vi "YokoGS200 Set Levelold.vi"(8 "error in (no error)":errorcluster, 9 "Auto Range":bool, 10 "Output Level":dbl min=-30.0 max=30.0 step=1e-08, 11 "VISA Rsrc":refnum<visa-resource-name>="SR530") -> (0 "error out":errorcluster, 3 "VISA Rsrc Out":refnum<visa-resource-name>="GPIB0::12::INSTR")   [LabVIEW 2012]
uses:
  <userlib>/Yoko GS200/YokoGS200 lvl_states ctl.ctl
panel:
  out "Octet d'état":bool[](array[boolean])
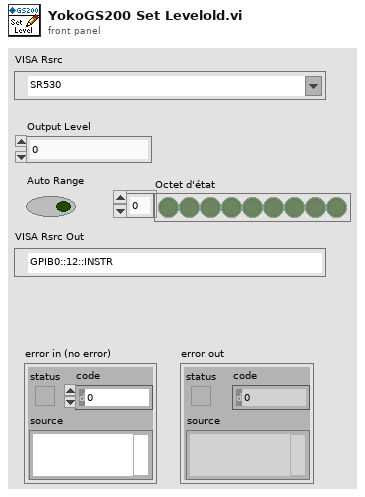
[diagram p1: front panel]
types:
  T1 = typedef "YokoGS200 lvl_states ctl.ctl" = enum16{"Send Command", "Check Errors", "End"}
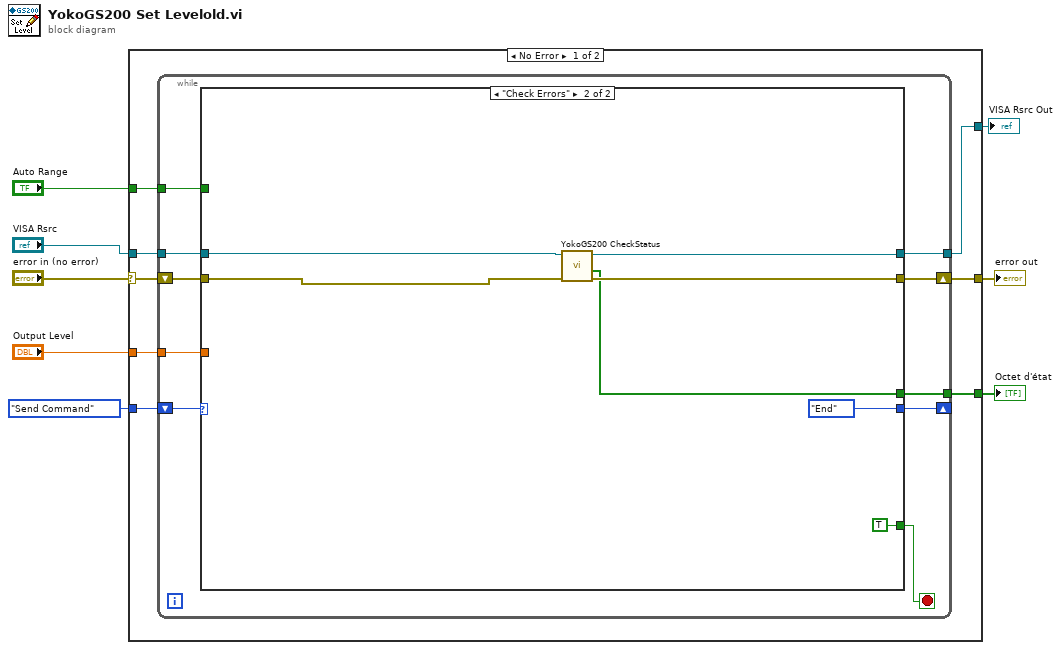
[diagram p0: block diagram]
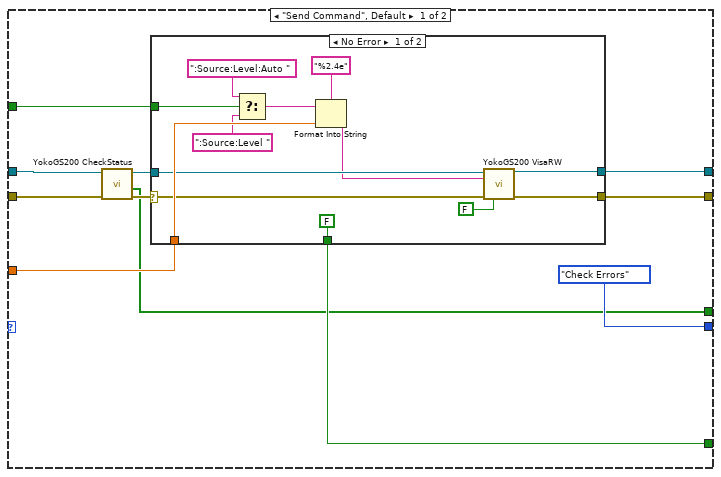
[diagram p2: hidden frame]
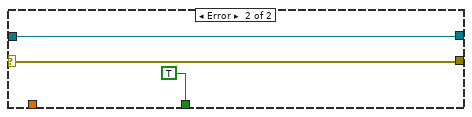
[diagram p3: hidden frame]
diagram:
  n1 = case shown="No Error" "error in (no error)" {
    selector: "error in (no error)" -> [w16 w61]
    tunnel: "VISA Rsrc" -> [w15 w62]
    tunnel: [w10 w61] -> w6
    tunnel: [w14 w62] -> w5
    tunnel: "Output Level" -> [w13 _]
    tunnel: "Auto Range" -> [w12 _]
    tunnel: YokoGS200_lvl_states_ctl."Send Command" ("Level State") -> [w11 _]
    tunnel: [w9 _] -> w1
    frame No Error {
      n2 = while {
        tunnel: w15 -> [w25]
        tunnel: [w24] -> w14
        tunnel: w13 -> [w23]
        tunnel: w12 -> [w22]
        shift-right: [w20] -> _
        shift-left: w11 -> [w21]
        shift-right: [w18] -> w10
        shift-left: w16 -> [w26]
        tunnel: [w17] -> w9
        stop <- w19 stop-if-true
        n3 = case shown="\"Check Errors\"" w21 {
          tunnel: w26 -> [w32 w54]
          tunnel: w25 -> [w31 w55]
          tunnel: [w37 w57] -> w24
          tunnel: w23 -> [w36 _]
          tunnel: [w34 w59] -> w18
          tunnel: w22 -> [w35 _]
          tunnel: [YokoGS200_lvl_states_ctl."Check Errors" ("Level State") YokoGS200_lvl_states_ctl."End" ("Level State")] -> w20
          tunnel: [w28 TRUE] -> w19
          tunnel: [w27 w56] -> w17
          frame "Send Command", Default {
            n4 = call <userlib>:"YokoGS200 CheckStatus.vi"("error in (no error)"=w32, "VISA Rsrc"=w31) -> ("error out"=w29:errorcluster, "Octet d'état"=w27:bool[], "VISA Rsrc Out"=w30:refnum<visa-resource-name>)  [unwired: 6 in, 1 out]
            n5 = case shown="No Error" w29 {
              selector: w29 -> [w41 w52]
              tunnel: [w50 w51] -> w37
              tunnel: w36 -> [w49 _]
              tunnel: w35 -> [w47 _]
              tunnel: [w43 w52] -> w34
              tunnel: w30 -> [w42 w51]
              tunnel: [FALSE TRUE] -> w28
              frame No Error {
                n6 = Select(t=":Source:Level:Auto " ("initial string"), s=w47, f=":Source:Level " ("initial string")) -> (s? t:f=w44:string)
                n7 = Format Into String(format string="%2.4e", initial string=w44, w49) -> (resulting string=w39:string)  [unwired: 1 in, 1 out]
                n8 = call <userlib>:"YokoGS200 VisaRW.vi"("VISA Rsrc"=w42, "ChaineCom"=w39, "error in (no error)"=w41, "Lecture?(T)"=FALSE) -> ("VISA Rsrc Out"=w50:refnum<visa-resource-name>, "error out"=w43:errorcluster)  [unwired: 7 in, 3 out]
              }
              frame Error {
              }
            }
          }
          frame "Check Errors" {
            n9 = call <userlib>:"YokoGS200 CheckStatus.vi"("error in (no error)"=w54, "VISA Rsrc"=w55) -> ("error out"=w59:errorcluster, "Octet d'état"=w56:bool[], "VISA Rsrc Out"=w57:refnum<visa-resource-name>)  [unwired: 6 in, 1 out]
          }
        }
      }
    }
    frame Error {
    }
  }
  "error out" <- w6
  "VISA Rsrc Out" <- w5
  "Octet d'état" <- w1
